vi "Palette Grid.vi"(11 "Positions":cluster{"Left":i32, "Top":i32}[](array[cluster])) -> (2 "Indexes":i32[][](array[numeric]), 3 "Label Index":i32)   [LabVIEW 2021, in "Markdown.lvlib"]
doc: "Returns the VI Tree palette positions based on the decorations. This calculates the grid positions by alignment on the VI Tree block dragram."
uses:
  Markdown.lvlib
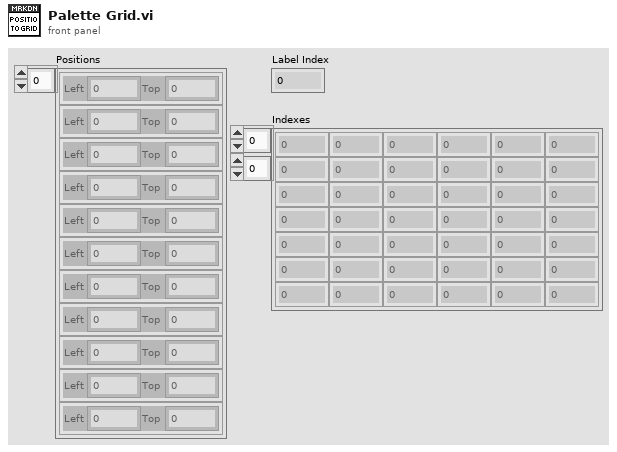
[diagram p1: front panel]
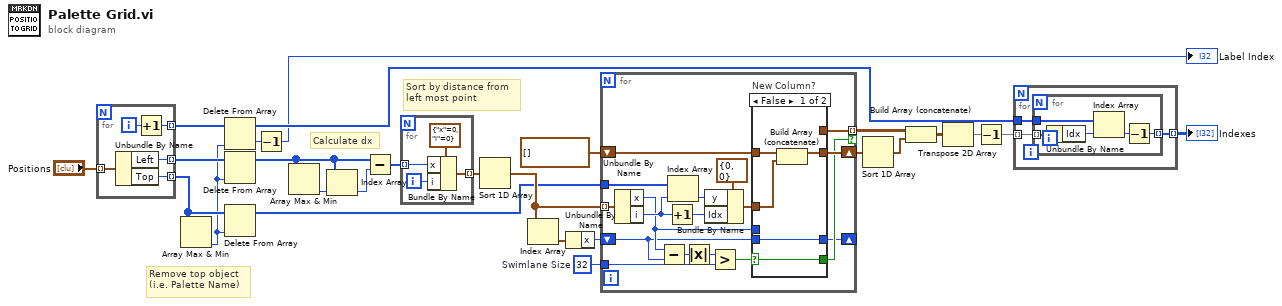
[diagram p0: block diagram]
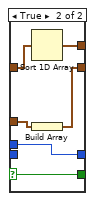
[diagram p2: hidden frame]
diagram:
  w26 = 32  # Swimlane Size
  # "Remove top object\n(i.e. Palette Name)"
  # "Calculate dx"
  # "Sort by distance from\nleft most point"
  n1 = for {
    tunnel: "Positions" -> [w31] mode=indexing
    tunnel: [w30] -> w13 mode=indexing
    tunnel: [w29] -> w14 mode=indexing
    tunnel: [w27] -> w12 mode=indexing
    i -> [w28]
    n2 = Unbundle By Name(w31) -> ("Left"=w29:i32, "Top"=w30:i32)
    n3 = Increment(x=w28) -> (x+1=w27:i32)
  }
  n4 = Array Max & Min(array=w13) -> (min index (indices)=w11:i32)  [unwired: 3 out]
  n5 = Delete From Array(array=w12, index=w11) -> (deleted portion=w2:i32, array with subset deleted=w4:i32[])  [unwired: 1 in]
  n6 = Delete From Array(array=w14, index=w11) -> (array with subset deleted=w8:i32[])  [unwired: 1 in, 1 out]
  n7 = Delete From Array(array=w13, index=w11) -> (array with subset deleted=w5:i32[])  [unwired: 1 in, 1 out]
  n8 = Decrement(x=w2) -> (x-1=→"Label Index":i32)
  n9 = Array Max & Min(array=w8) -> (min index (indices)=w9:i32)  [unwired: 3 out]
  n10 = Index Array(array=w8, index=w9) -> (element=w10:i32)
  n11 = Subtract(x=w8, y=w10) -> (x-y=w7:i32[])
  n12 = for {
    tunnel: w7 -> [w35] mode=indexing
    tunnel: [w34] -> w6 mode=indexing
    i -> [w32]
    n13 = Bundle By Name(cluster=cluster{"x":i32, "i":i32} {"x"=0, "i"=0} ("SortX"), "x"=w35, "i"=w32) -> (w34:cluster{"x":i32, "i":i32})
  }
  n14 = Sort 1D Array(array=w6) -> (sorted array=w25:cluster{"x":i32, "i":i32}[])
  n15 = Index Array(array=w25) -> (element=w24:cluster{"x":i32, "i":i32})  [unwired: 1 in]
  n16 = Unbundle By Name(w24) -> ("x"=w23:i32)
  n17 = for {
    tunnel: w25 -> [w36] mode=indexing
    tunnel: w26 -> [w53]
    shift-right: [w47] -> _
    shift-left: w23 -> [w40]
    shift-right: [w51] -> w19
    shift-left: cluster{"y":i32, "Idx":i32}[] [] -> [w52]
    tunnel: [w49] -> w21 mode=indexing if=w48
    tunnel: w5 -> [w45]
    n18 = Unbundle By Name(w36) -> ("x"=w41:i32, "i"=w43:i32)
    n19 = Subtract(x=w41, y=w40) -> (x-y=w39:i32)
    n20 = Increment(x=w43) -> (x+1=w42:i32)
    n21 = Index Array(array=w45, index=w43) -> (element=w44:i32)
    n22 = Absolute Value(x=w39) -> (abs(x)=w38:i32)
    n23 = Bundle By Name(cluster=cluster{"y":i32, "Idx":i32} {"y"=0, "Idx"=0} ("SortY"), "y"=w44, "Idx"=w42) -> (w46:cluster{"y":i32, "Idx":i32})
    n24 = Greater?(x=w38, y=w53) -> (0:w50:bool)
    n25 = case "New Column?" shown="False" w50 {
      selector: w50 -> [w54 w59]
      tunnel: w52 -> [w58 w60]
      tunnel: w46 -> [w57 w64]
      tunnel: [w56 w63] -> w51
      tunnel: w41 -> [_ w62]
      tunnel: w40 -> [w55 _]
      tunnel: [_ w61] -> w49
      tunnel: [w54 w59] -> w48
      tunnel: [w55 w62] -> w47
      frame False {
        n26 = Build Array (concatenate)(w58, w57) -> (w56:cluster{"y":i32, "Idx":i32}[])
      }
      frame True {
        n27 = Sort 1D Array(array=w60) -> (sorted array=w61:cluster{"y":i32, "Idx":i32}[])
        n28 = Build Array(w64) -> (w63:cluster{"y":i32, "Idx":i32}[])
      }
    }
  }
  n29 = Sort 1D Array(array=w19) -> (sorted array=w18:cluster{"y":i32, "Idx":i32}[])
  n30 = Build Array (concatenate)(w21, w18) -> (w17:cluster{"y":i32, "Idx":i32}[][])
  n31 = Transpose 2D Array(2D array=w17) -> (transposed array=w16:cluster{"y":i32, "Idx":i32}[][])
  n32 = Decrement(x=w16) -> (x-1=w20:cluster{"y":i32, "Idx":i32}[][])
  n33 = for {
    tunnel: w20 -> [w67] mode=indexing
    tunnel: w4 -> [w66]
    tunnel: [w65] -> w3 mode=indexing
    n34 = for {
      tunnel: w67 -> [w72] mode=indexing
      tunnel: w66 -> [w71]
      tunnel: [w68] -> w65 mode=indexing
      n35 = Unbundle By Name(w72) -> ("Idx"=w70:i32)
      n36 = Index Array(array=w71, index=w70) -> (element=w69:i32)
      n37 = Decrement(x=w69) -> (x-1=w68:i32)
    }
  }
  "Indexes" <- w3
